vi "Test -- INI Creation.vi"() -> ()   [LabVIEW 2013]
uses:
  source/Manager.Text.INI/ConfigManager.Text.INI.lvclass
  source/Manager/Decompose KVPs.vi
  source/Manager/Write.vi
  source/Manager/ConfigManager.lvclass
  source/Manager.Text/ConfigManager.Text.lvclass
panel:
  out "Config":T1={"String"="test", "Numeric"=3.14159, "Boolean"=TRUE}
  out "text":string
  out "error out":errorcluster
  out "filepath":path
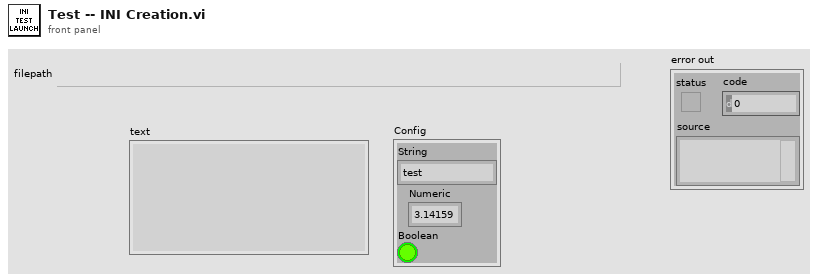
[diagram p1: front panel]
types:
  T1 = cluster{"String":string, "Numeric":dbl, "Boolean":bool}
  T2 = enum16{"open", "replace", "create", "open or create", "replace or create", "replace or create with confirmation"}
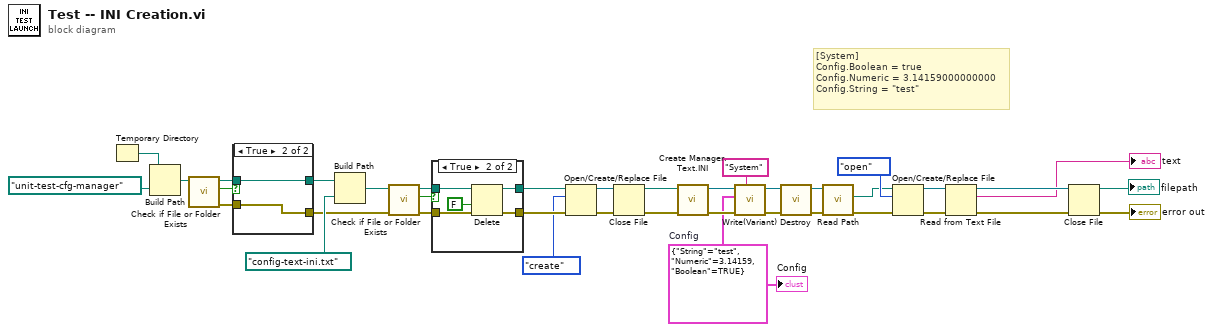
[diagram p0: block diagram]
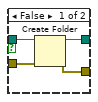
[diagram p3: hidden frame]
diagram:
  w29 = T1 {"String"="test", "Numeric"=3.14159, "Boolean"=TRUE}  # Config
  # "[System]\nConfig.Boolean = true\nConfig.Numeric = 3.14159000000000\nConfig.String = \"test\""
  n1 = Temporary Directory() -> (w36:path)
  n2 = Build Path(base path=w36, name or relative path=path "unit-test-cfg-manager") -> (appended path=w34:path)
  n3 = call <vilib>:"Check if File or Folder Exists.vi"("path"=w34) -> ("error out"=w23:errorcluster, "file or folder exists?"=w32:bool, "dup path"=w33:path)  [unwired: 8 in]
  n4 = case shown="True" w32 {
    tunnel: w33 -> [w41 w43]
    tunnel: [w40 w43] -> w28
    tunnel: w23 -> [w39 w42]
    tunnel: [w38 w42] -> w18
    frame False {
      n5 = Create Folder(path (use dialog)=w41, error in=w39) -> (created path=w40:path, error out=w38:errorcluster)  [unwired: 1 in, 1 out]
    }
    frame True {
    }
  }
  n6 = Build Path(base path=w28, name or relative path=path "config-text-ini.txt" ("filepath 2")) -> (appended path=w22:path)
  n7 = call <vilib>:"Check if File or Folder Exists.vi"("error in (no error)"=w18, "path"=w22) -> ("error out"=w20:errorcluster, "file or folder exists?"=w19:bool, "dup path"=w21:path)  [unwired: 7 in]
  n8 = case shown="True" w19 {
    tunnel: [w45 w49] -> w12
    tunnel: w21 -> [w45 w48]
    tunnel: w20 -> [w44 w47]
    tunnel: [w44 w46] -> w15
    frame False {
    }
    frame True {
      n9 = Delete(path (use dialog)=w48, confirm (F)=FALSE, error in=w47) -> (deleted path=w49:path, error out=w46:errorcluster)  [unwired: 2 in, 1 out]
    }
  }
  n10 = Open/Create/Replace File(file path (use dialog)=w12, error in=w15, operation (0:open)=T2."create") -> (refnum out=w14:refnum<file>, error out=w17:errorcluster)  [unwired: 3 in, 1 out]
  n11 = Close File(refnum=w14, error in=w17) -> (path=w13:path, error out=w16:errorcluster)
  n12 = call "Create Manager.Text.INI.vi"("error in (no error)"=w16, "filepath"=w13) -> ("error out"=w30:errorcluster, "ConfigManager.Text.INI out"=w31:refnum<class "ConfigManager.Text.INI.lvclass">)  [unwired: 7 in, 1 out]
  n13 = call "Write(Variant).vi"("Qualified Name"="System", "error in (no error)"=w30, "value"=w29, "ConfigManager in"=w31) -> ("error out"=w25:errorcluster, "ConfigManager out"=w26:refnum<class "ConfigManager.Text.INI.lvclass">)  [unwired: 5 in, 1 out]
  n14 = call-dynamic "Destroy.vi"("error in (no error)"=w25, "ConfigManager.Text in"=w26) -> ("error out"=w7:errorcluster, "ConfigManager.Text out"=w24:refnum<class "ConfigManager.Text.INI.lvclass">)  [unwired: 8 in]
  n15 = call "Read Path.vi"("ConfigManager.Text in"=w24) -> ("Path"=w9:path)  [unwired: 9 in, 1 out]
  n16 = Open/Create/Replace File(file path (use dialog)=w9, error in=w7, operation (0:open)=T2."open") -> (refnum out=w5:refnum<file>, error out=w3:errorcluster)  [unwired: 3 in, 1 out]
  n17 = Read from Text File(file (use dialog)=w5, error in=w3) -> (refnum out=w4:refnum<file>, text=→"text":string, error out=w2:errorcluster)  [unwired: 2 in, 1 out]
  n18 = Close File(refnum=w4, error in=w2) -> (path=→"filepath":path, error out=→"error out":errorcluster)
  "Config" <- w29
